vi "ERDWrite_To_GEA2.vi"() -> ()   [LabVIEW 2016]
uses:
  type defs/ERD Write Data In.ctl
  type defs/Data Type.ctl
  type defs/Source_Destination.ctl
  library/GEA2_Toolkit.lvlib
panel:
  out "Error Out":errorcluster
  in  "Error In":errorcluster
  out "GEA2 Message Data":T1 {"ERD Number" format="%.0x"}
  in  "GEA Inputs":T3 {"Destination" format="%.0x"; "Source" format="%.0x"}
  in  "Write ERD List":T1[](array[typedef]) {"ERD Number" format="%.0x"}
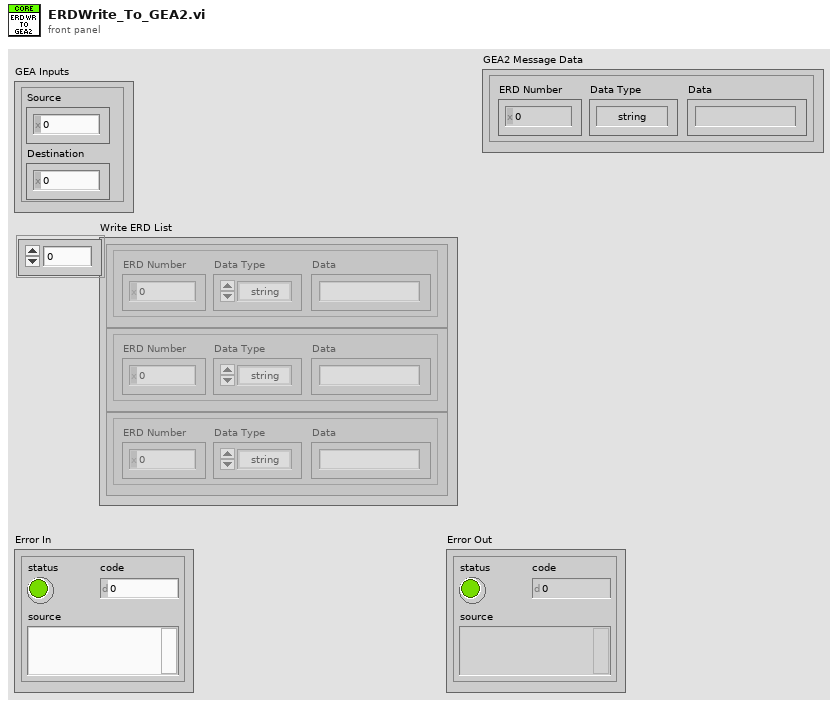
[diagram p1: front panel]
types:
  T1 = typedef "GEA2_Toolkit.lvlib/ERD Write Data In.ctl" = cluster{"ERD Number":u16, "Data Type":T2, "Data":string}
  T2 = typedef "GEA2_Toolkit.lvlib/Data Type.ctl" = enum16{"string", "boolean", "uint8_t", "uint16_t", "uint32_t", "uint64_t"}
  T3 = typedef "GEA2_Toolkit.lvlib/Source_Destination.ctl" = cluster{"Source":u8, "Destination":u8}
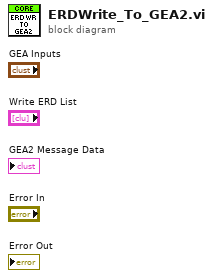
[diagram p0: block diagram]
diagram:
